vi "libssh2_sftp_open_ex.vi"(5 "open_type (0 = file)":i32(ring) items=["File", "Directory"], 7 "mode":i32(ring) items=["LIBSSH2_SFTP_S_IRWXU"=448, "LIBSSH2_SFTP_S_IRUSR"=256, "LIBSSH2_SFTP_S_IWUSR"=128, "LIBSSH2_SFTP_S_IXUSR"=64, "LIBSSH2_SFTP_S_IRWXG"=56, "LIBSSH2_SFTP_S_IRGRP"=32, "LIBSSH2_SFTP_S_IWGRP"=16, "LIBSSH2_SFTP_S_IXGRP"=8, "LIBSSH2_SFTP_S_IRWXO"=7, "LIBSSH2_SFTP_S_IROTH"=4, "LIBSSH2_SFTP_S_IWOTH"=2, "LIBSSH2_SFTP_S_IXOTH"=1], 8 "error in (no error)":errorcluster, 9 "flags":u32(ring) format="%x" items=["LIBSSH2_FXF_READ"=1, "LIBSSH2_FXF_WRITE"=2, "LIBSSH2_FXF_APPEND"=4, "LIBSSH2_FXF_CREAT"=8, "LIBSSH2_FXF_TRUNC"=16, "LIBSSH2_FXF_EXCL"=32], 10 "filename":string, 11 "sftp":T2) -> (0 "error out":errorcluster, 3 "sftp handle":T1)   [LabVIEW 2017, in "libssh2.lvlib"]
doc: "Open a file or directory handle with custom flags and permissions."
uses:
  libssh2.lvlib
  SFTP Refnum.ctl
  SFTP Handle Refnum.ctl
  Acquire Session.vi
  Release Session.vi
  Not An SFTP Refnum.vi
  <vilib>/Utility/error.llb/Error Cluster From Error Code.vi
  Global Settings.vi
  Read SFTP Refnum.vi
  Read Session Refnum.vi
  <vilib>/Utility/semaphor.llb/Acquire Semaphore.vi
  <vilib>/Utility/semaphor.llb/Release Semaphore.vi
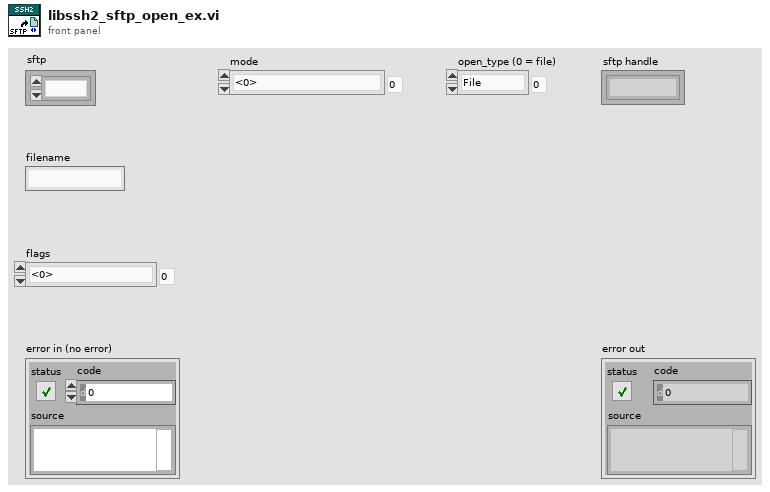
[diagram p1: front panel]
types:
  T1 = typedef "libssh2.lvlib/SFTP Handle Refnum.ctl" = refnum<k1>
  T2 = typedef "libssh2.lvlib/SFTP Refnum.ctl" = refnum<k1>
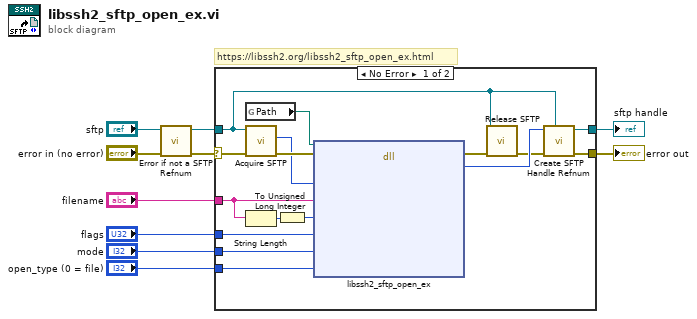
[diagram p0: block diagram]
diagram:
  # "https://libssh2.org/libssh2_sftp_open_ex.html"
  n1 = call "Error if not a SFTP Refnum.vi"("error in (no error)"="error in (no error)", "sftp"="sftp") -> ("error out"=w9:errorcluster, "sftp out"=w8:T2)  [unwired: 8 in]
  n2 = case shown="No Error" w9 {
    selector: w9 -> [w25 w27]
    tunnel: w8 -> [w11 _]
    tunnel: [w21 w27] -> w7
    tunnel: [w19 _] -> w1
    tunnel: "filename" -> [w18 _]
    tunnel: "flags" -> [w15 _]
    tunnel: "mode" -> [w14 _]
    tunnel: "open_type (0 = file)" -> [w13 _]
    frame No Error {
      n3 = global read "Global Settings.vi" "Path"() -> (w26:path)
      n4 = call "Acquire SFTP.vi"("error in (no error)"=w25, "sftp"=w11) -> ("error out"=w24:errorcluster, "LIBSSH2_SFTP*"=w23:u64)  [unwired: 8 in]
      n5 = String Length(string=w18) -> (length=w17:i32)
      n6 = To Unsigned Long Integer(number=w17) -> (unsigned 32bit integer=w16:u32)
      n7 = dll-call lib="?" fn="libssh2_sftp_open_ex"(path in=w26, error in=w24, "sftp"=w23, "filename"=w18, "filename_len"=w16, "flags"=w15, "mode"=w14, "open_type"=w13) -> (error out=w22:errorcluster, "return value"=w20:u64)  [unwired: 7 in, 1 out]
      n8 = call "Release SFTP.vi"("error in (no error)"=w22, "sftp"=w11) -> ("error out"=w12:errorcluster)  [unwired: 9 in]
      n9 = call "Create SFTP Handle Refnum.vi"("sftp"=w11, "error in (no error)"=w12, "LIBSSH2_SFTP_HANDLE*"=w20) -> ("error out"=w21:errorcluster, "sftp handle"=w19:T1)  [unwired: 7 in]
    }
    frame Error {
    }
  }
  "error out" <- w7
  "sftp handle" <- w1
